vi "Subvi debouncer.vi"(1 "Input":bool, 3 "CyclesToFilter_tick":u32) -> (8 "Output":bool)   [LabVIEW 2017]
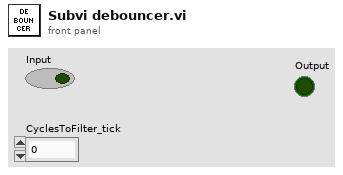
[diagram p1: front panel]
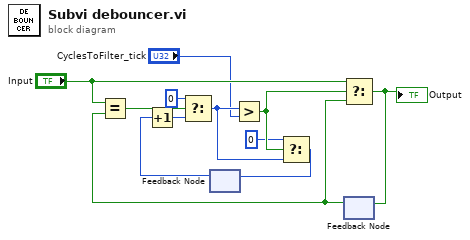
[diagram p0: block diagram]
diagram:
  n1 = feedback #1() -> (w5:u32)  [unwired: 1 in]
  n2 = Increment(x=w5) -> (x+1=w6:u32)
  n3 = feedback #2() -> (w2:bool)  [unwired: 1 in]
  n4 = Equal?(x="Input", y=w2) -> (x = y?=w10:bool)
  n5 = Select(t=u32 0, s=w10, f=w6) -> (s? t:f=w4:u32)
  n6 = Greater?(x=w4, y="CyclesToFilter_tick") -> (0:w8:bool)
  n7 = Select(t=u32 0, s=w8, f=w4) -> (s? t:f=w12:u32)
  n8 = feedback-in #1(w12) -> ()
  n9 = Select(t="Input", s=w8, f=w2) -> (s? t:f=w3:bool)
  "Output" <- w3
  n10 = feedback-in #2(w3) -> ()
